vi "AutoCheap.vi"(8 "error in":errorcluster) -> ()   [LabVIEW 2014]
uses:
  AutomationGlobals.vi
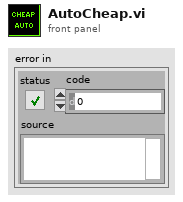
[diagram p1: front panel]
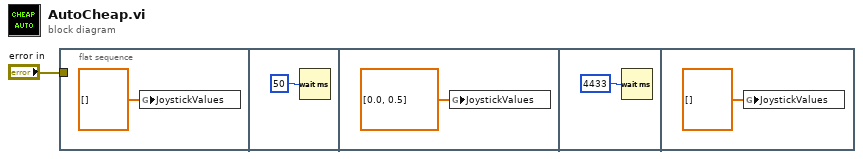
[diagram p0: block diagram]
diagram:
  n1 = flat-sequence {
    tunnel: "error in" -> [_]
    frame #0 {
      n2 = global write "AutomationGlobals.vi" "JoystickValues"(dbl[] [] ("s? t:f")) -> ()
    }
    frame #1 {
      n3 = Wait (ms)(milliseconds to wait=u32 50) -> ()  [unwired: 1 out]
    }
    frame #2 {
      n4 = global write "AutomationGlobals.vi" "JoystickValues"(dbl[] [0.0, 0.5] ("s? t:f")) -> ()
    }
    frame #3 {
      n5 = Wait (ms)(milliseconds to wait=u32 4433) -> ()  [unwired: 1 out]
    }
    frame #4 {
      n6 = global write "AutomationGlobals.vi" "JoystickValues"(dbl[] [] ("s? t:f")) -> ()
    }
  }
